vi "find_output.vi"(6 "find output":dbl format="%.4p", 8 "output 2":dbl format="%.4p", 9 "output 1":dbl format="%.4p", 10 "input 2":dbl format="%.4p", 11 "input 1":dbl format="%.4p") -> (3 "getInput":dbl format="%.4p")   [LabVIEW 2014]
panel:
  in  "m":dbl format="%.4p"
  out "eðim":dbl format="%.4p"
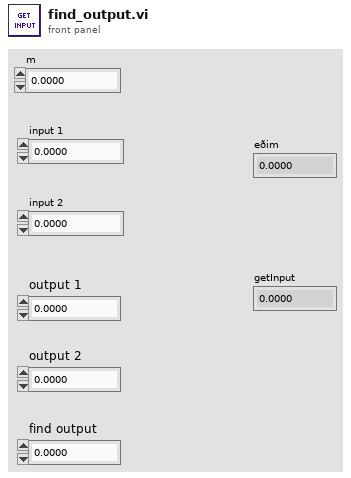
[diagram p1: front panel]
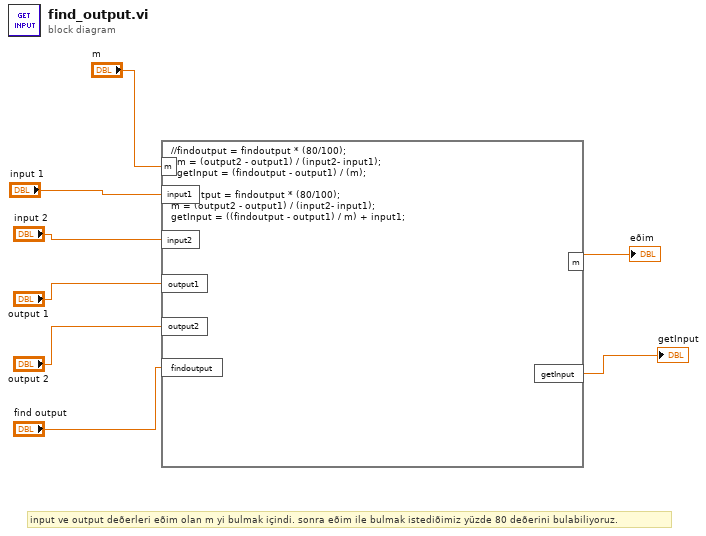
[diagram p0: block diagram]
diagram:
  # "input ve output deðerleri eðim olan m yi bulmak içindi. sonra eðim ile bulmak istediðimiz yüzde 80 deðerini bulabiliyoruz."
  n1 = formula code="//findoutput = findoutput * (80/100);\n//m = (output2 - output1) / (input2- input1);\n//getInput = (findoutput - output1) / (m);\n\nfindoutput = findoutput * (80/100);\nm = (output2 - output1) / (input2- input1);\ngetInput = ((findoutput - output1) / m) + input1;"("input1"="input 1", "input2"="input 2", "output1"="output 1", "output2"="output 2", "findoutput"="find output", "m"="m") -> ("getInput"=→"getInput":dbl, "m"=→"eðim":dbl)
